vi "Add-Ex-Mod-Manualy-SSA.vi"(8 "In-Ex_Mod_IDs":string[](array[string])=["LacI", "TetR"], 9 "In-Idx of Mod in Sp IDs":i32[](array[numeric]), 11 "Sp IDs":string[](array[string])) -> (1 "Out-Ex_Mod_IDs":string[](array[string])=["LacI", "TetR"], 2 "O/p Idx of Mod in Sp IDs":i32[](array[numeric])=[1, 4])   [LabVIEW 2014]
doc: "This VI is used to select the name of species which a user wants to make the external controls of. \n\nDesigned by:\nHB\nhaba@dtu.dk"
panel:
  in  "Done":bool
  in  "Make external controls of:":i32(listbox)
  in  "Available species:":i32(listbox)
  # "Select species for external controls"
  # "Drag the name of species from left-hand box and drop it to right-hand box."
  # "-->"
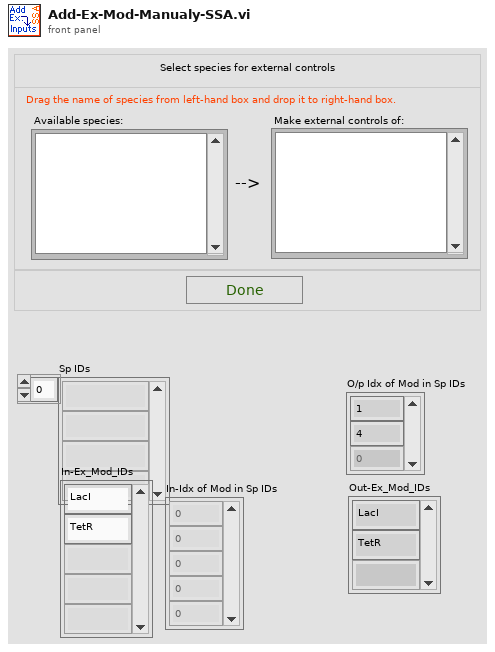
[diagram p1: front panel]
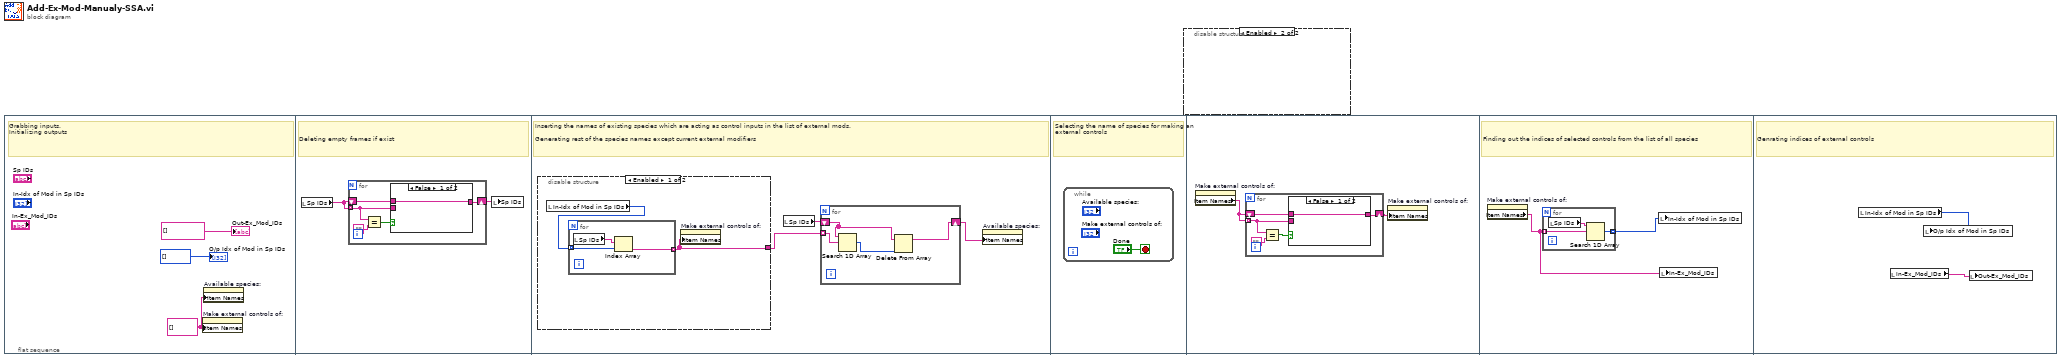
[diagram p0: block diagram]
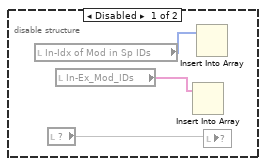
[diagram p2: hidden frame]
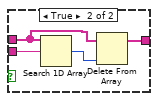
[diagram p3: hidden frame]
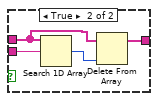
[diagram p5: hidden frame]
diagram:
  n1 = flat-sequence {
    frame #0 {
      w1 = string[] [] ("Item Names")
      # "Grabbing inputs. \nInitializing outputs"
      n2 = property on="Make external controls of:" class="LstBox (strict)"("Item Names"=w1) -> ()  [unwired: 2 in, 2 out]
      n3 = property on="Available species:" class="LstBox (strict)"("Item Names"=w1) -> ()  [unwired: 2 in, 2 out]
      "O/p Idx of Mod in Sp IDs" <- i32[] [] ("O/p Idx of Mod in Sp IDs")
      "Out-Ex_Mod_IDs" <- string[] [] ("Ex_Mod_IDs")
    }
    frame #1 {
      # "Deleting empty frames if exist"
      n4 = local read "Sp IDs"() -> (w5:string[])
      n5 = for {
        shift-right: [w6] -> w4
        shift-left: w5 -> [w8]
        tunnel: w5 -> [w7] mode=indexing
        n6 = Equal?(x=w7, y="") -> (x = y?=w9:bool)
        n7 = case shown="False" w9 {
          tunnel: w8 -> [w11 w14]
          tunnel: w7 -> [_ w13]
          tunnel: [w11 w12] -> w6
          frame False {
          }
          frame True {
            n8 = Search 1D Array(1D array=w14, element=w13) -> (index of element=w15:i32)  [unwired: 1 in]
            n9 = Delete From Array(array=w14, index=w15) -> (array with subset deleted=w12:string[])  [unwired: 1 in, 1 out]
          }
        }
      }
      n10 = local write "Sp IDs"(w4) -> ()
    }
    frame #2 {
      # "Inserting the names of existing species which are acting as control inputs in the list of external mods.\n\nGenerating rest of the species names except current external modifiers"
      n11 = disable-structure shown="Enabled" {
        disable-tunnel: [w23 _] -> w18
        frame Enabled {
          n12 = local read "In-Idx of Mod in Sp IDs"() -> (w24:i32[])
          n13 = for {
            tunnel: w24 -> [w25] mode=indexing
            tunnel: [w26] -> w23 mode=indexing
            n14 = local read "Sp IDs"() -> (w27:string[])
            n15 = Index Array(array=w27, index=w25) -> (element=w26:string)
          }
          n16 = property on="Make external controls of:" class="LstBox (strict)"("Item Names"=w23) -> ()  [unwired: 2 in, 2 out]
        }
        frame Disabled {
        }
      }
      n17 = local read "Sp IDs"() -> (w17:string[])
      n18 = for {
        tunnel: w18 -> [w22] mode=indexing
        shift-right: [w19] -> w16
        shift-left: w17 -> [w20]
        n19 = Search 1D Array(1D array=w20, element=w22) -> (index of element=w21:i32)  [unwired: 1 in]
        n20 = Delete From Array(array=w20, index=w21) -> (array with subset deleted=w19:string[])  [unwired: 1 in, 1 out]
      }
      n21 = property on="Available species:" class="LstBox (strict)"("Item Names"=w16) -> ()  [unwired: 2 in, 2 out]
    }
    frame #3 {
      # "Selecting the name of species for making an external controls"
      n22 = while {
        stop <- "Done" stop-if-true
      }
    }
    frame #4 {
      n23 = property on="Make external controls of:" class="LstBox (strict)"() -> ("Item Names"=w30:string[])  [unwired: 2 in, 2 out]
      n24 = for {
        shift-right: [w31] -> w29
        shift-left: w30 -> [w33]
        tunnel: w30 -> [w32] mode=indexing
        n25 = Equal?(x=w32, y="") -> (x = y?=w34:bool)
        n26 = case shown="False" w34 {
          tunnel: w33 -> [w36 w39]
          tunnel: w32 -> [_ w38]
          tunnel: [w36 w37] -> w31
          frame False {
          }
          frame True {
            n27 = Search 1D Array(1D array=w39, element=w38) -> (index of element=w40:i32)  [unwired: 1 in]
            n28 = Delete From Array(array=w39, index=w40) -> (array with subset deleted=w37:string[])  [unwired: 1 in, 1 out]
          }
        }
      }
      n29 = property on="Make external controls of:" class="LstBox (strict)"("Item Names"=w29) -> ()  [unwired: 2 in, 2 out]
    }
    frame #5 {
      # "Finding out the indices of selected controls from the list of all species"
      n30 = property on="Make external controls of:" class="LstBox (strict)"() -> ("Item Names"=w41:string[])  [unwired: 2 in, 2 out]
      n31 = for {
        tunnel: w41 -> [w45] mode=indexing
        tunnel: [w44] -> w42 mode=indexing
        n32 = local read "Sp IDs"() -> (w43:string[])
        n33 = Search 1D Array(1D array=w43, element=w45) -> (index of element=w44:i32)  [unwired: 1 in]
      }
      n34 = local write "In-Idx of Mod in Sp IDs"(w42) -> ()
      n35 = local write "In-Ex_Mod_IDs"(w41) -> ()
    }
    frame #6 {
      # "Genrating indices of external controls"
      n36 = local read "In-Idx of Mod in Sp IDs"() -> (w47:i32[])
      n37 = local read "In-Ex_Mod_IDs"() -> (w46:string[])
      n38 = local write "O/p Idx of Mod in Sp IDs"(w47) -> ()
      n39 = local write "Out-Ex_Mod_IDs"(w46) -> ()
    }
  }
  n40 = disable-structure shown="Enabled" {
    frame Disabled {
      n41 = local read "In-Idx of Mod in Sp IDs"() -> (w50:i32[])
      n42 = local read item#-1() -> (w48)
      n43 = local read "In-Ex_Mod_IDs"() -> (w49:string[])
      n44 = Insert Into Array(array=w49) -> ()  [unwired: 2 in, 1 out]
      n45 = Insert Into Array(array=w50) -> ()  [unwired: 2 in, 1 out]
      n46 = local write item#-1(w48) -> ()
    }
    frame Enabled {
    }
  }
